vi "main.vi"() -> ()   [LabVIEW 2021]
uses:
  Controls/App Data.ctl
  Controls/UI References.ctl
  <extravilib>/ChannelInstances/Stream-c(dbl,dbl)/Read With Abort.vi
  <extravilib>/ChannelInstances/Stream-c(dbl,dbl)/Write With Abort.vi
  <extravilib>/ChannelInstances/Stream-c(dbl,dbl)/EndpointRead.vi
  <extravilib>/ChannelInstances/Stream-c(dbl,dbl)/Endpoint.vi
  <extravilib>/ChannelInstances/Event Messenger-c(str,var)/Instantiate.vi
  <extravilib>/ChannelInstances/Event Messenger-c(str,var)/))Channel.vi
  <extravilib>/ChannelInstances/Stream-c(dbl,dbl)/Instantiate.vi
  <extravilib>/ChannelInstances/Stream-c(dbl,dbl)/)Channel.vi
  <resource>/ChannelSupport/_ChannelSupport/WaitIfNeeded.vi
  <vilib>/Instr/_visa.llb/VISA Configure Serial Port (Instr).vi
  <extravilib>/ChannelInstances/Stream-c(dbl,dbl).lvlib
  <extravilib>/ChannelInstances/Event Messenger-c(str,var).lvlib
panel:
  in  "Confirm":bool
  in  "Start":bool
  out "File Path":path
  out "Recording?":bool
  in  "Record?":bool
  out "XY Graph":cluster{"X":dbl, "Y":dbl}[](graph)
  out "Strain":dbl
  out "Time":dbl
  in  "VISA resource name":refnum<visa-resource-name>
  in  "Stop":bool
  # "Select the VISA resource name before starting the application, you can choose to record to a file at any time using the checkbox. Data acquisition begins after you press Start."
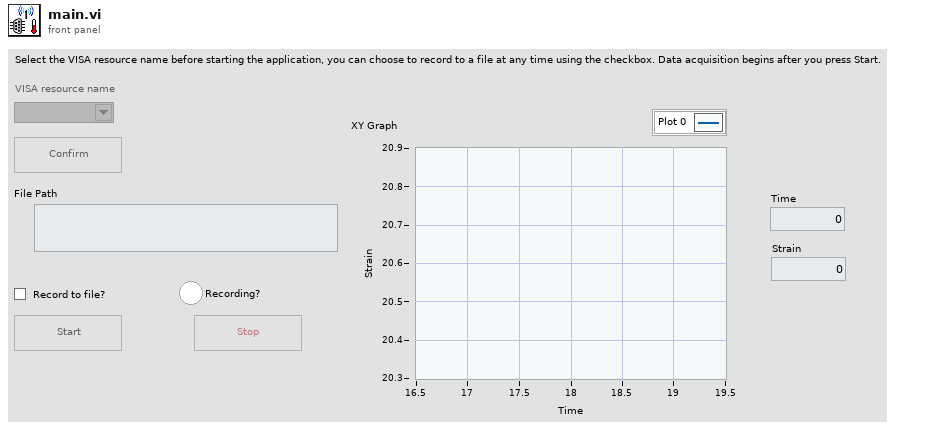
[diagram p1: front panel]
types:
  T1 = typedef "UI References.ctl" = cluster{"VISA resource name":refnum<vi>, "Confirm":refnum<vi>, "Start":refnum<vi>, "Stop":refnum<vi>, "Record?":refnum<vi>, "Recording?":refnum<vi>, "XY Graph":refnum<vi>}
  T2 = typedef "App Data.ctl" = cluster{"VISA resource name":refnum<visa-resource-name>, "File ref":refnum<file>}
  T3 = typedef "Event Messenger-c(str,var).lvlib/))Channel.ctl" = refnum<queue>
  T4 = typedef "Stream-c(dbl,dbl).lvlib/)Channel.ctl" = refnum<queue>
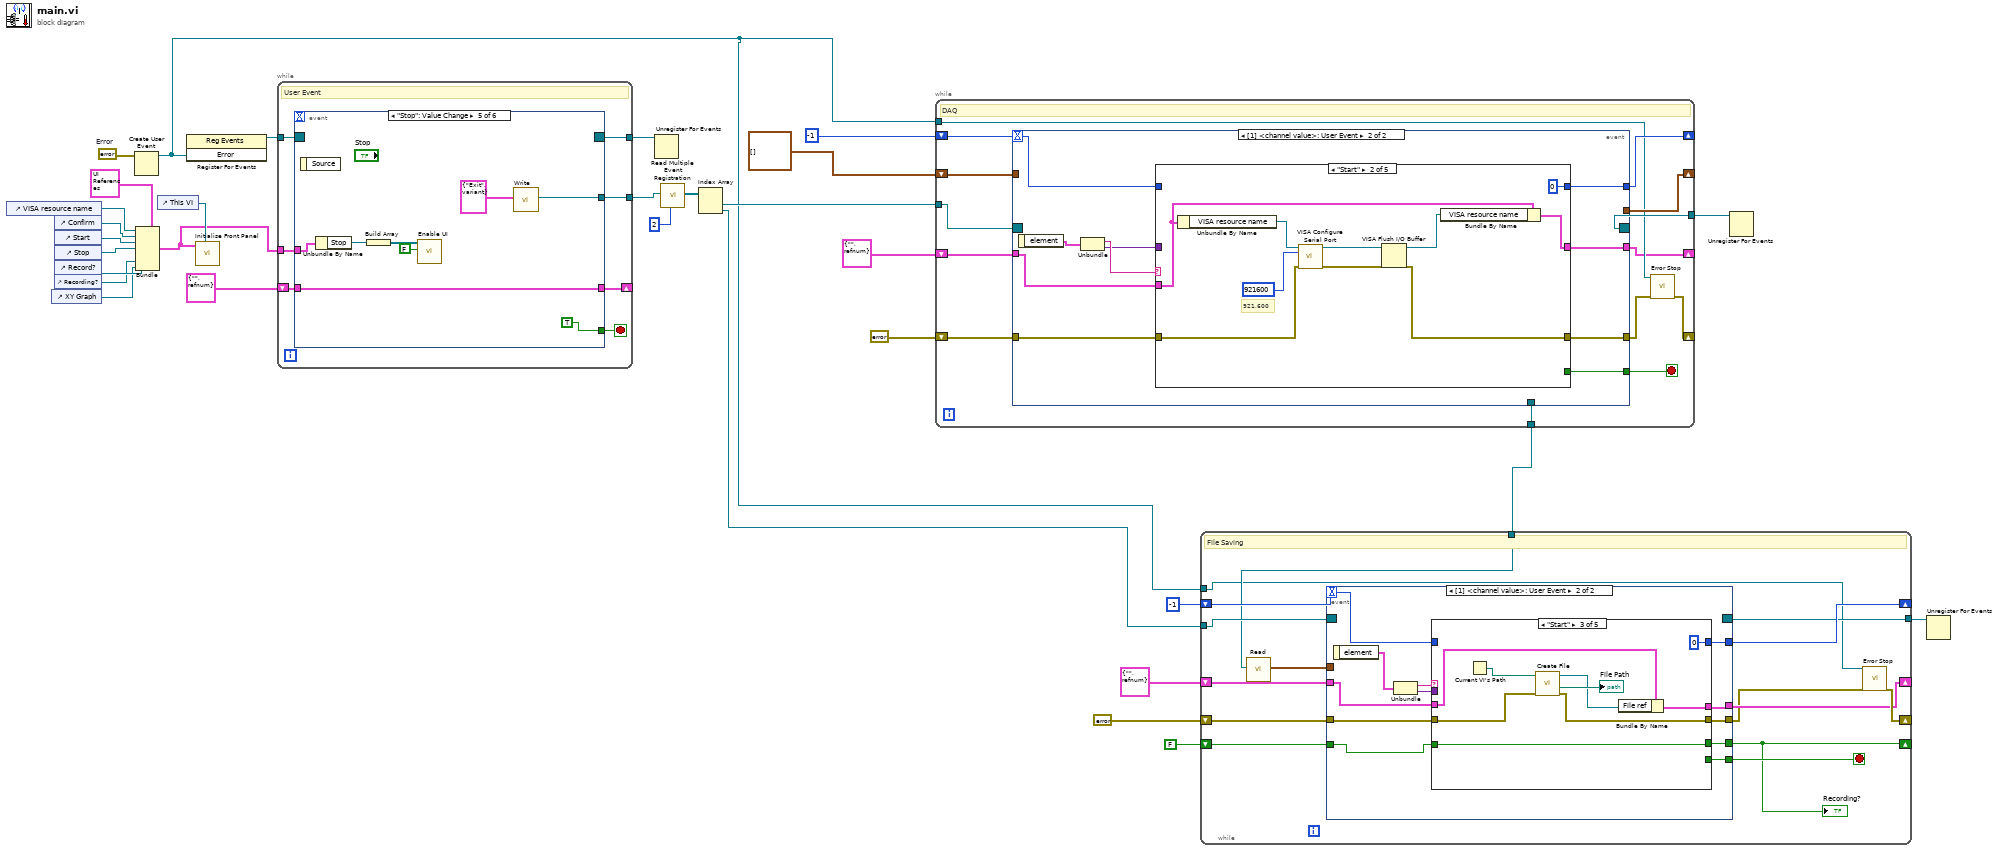
[diagram p0: block diagram]
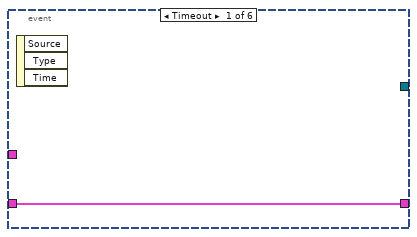
[diagram p2: hidden frame]
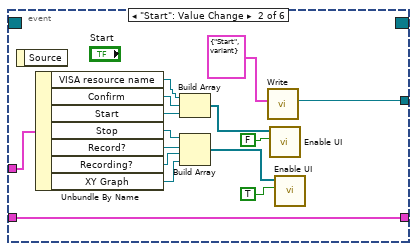
[diagram p3: hidden frame]
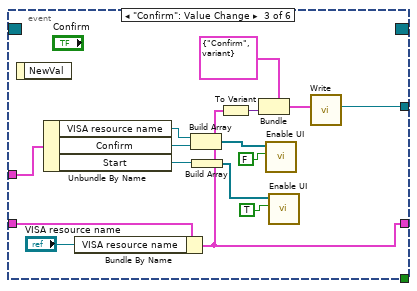
[diagram p4: hidden frame]
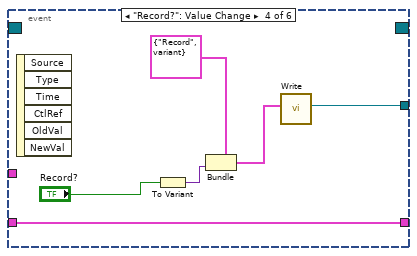
[diagram p5: hidden frame]
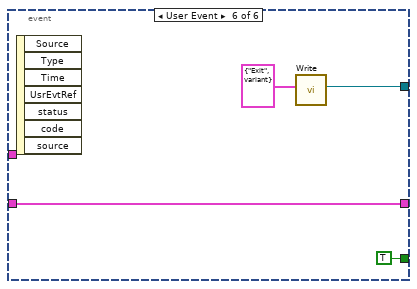
[diagram p6: hidden frame]
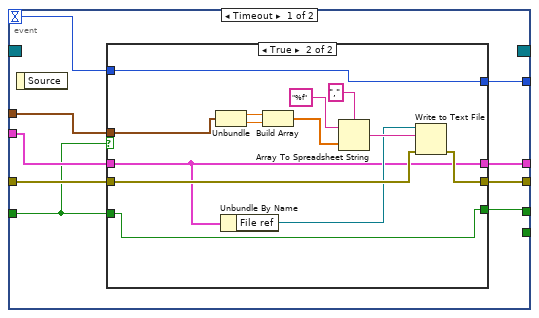
[diagram p7: hidden frame]
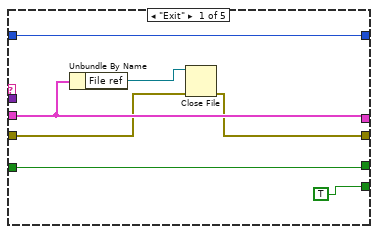
[diagram p9: hidden frame]
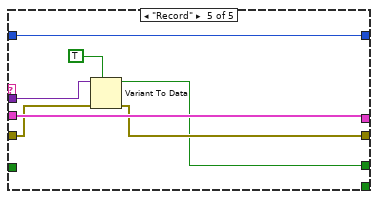
[diagram p12: hidden frame]
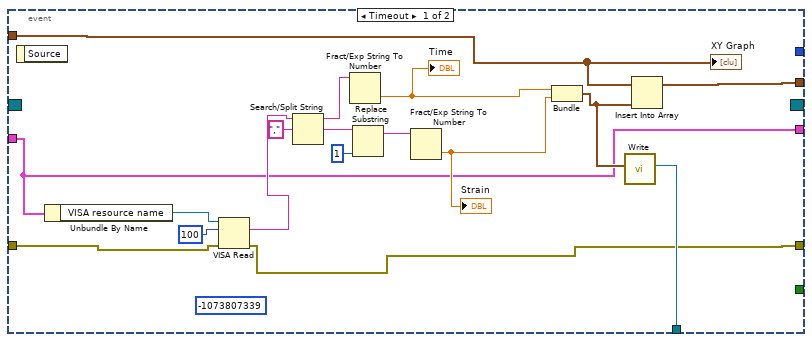
[diagram p13: hidden frame]
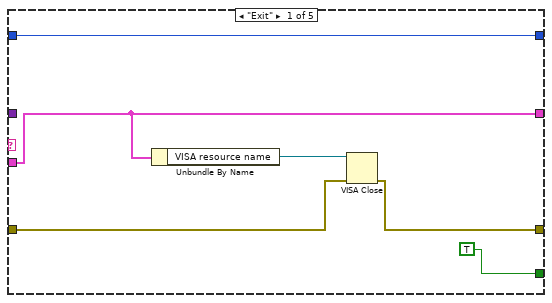
[diagram p14: hidden frame]
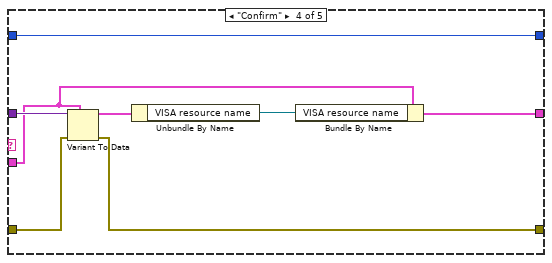
[diagram p16: hidden frame]
diagram:
  w23 = errorcluster {"status"=FALSE, "code"=0, "source"=""}  # Error
  n1 = control-ref of="VISA resource name"() -> (w4:refnum<vi>)
  n2 = control-ref of="XY Graph"() -> (w6:refnum<vi>)
  n3 = control-ref of="Confirm"() -> (w3:refnum<vi>)
  n4 = control-ref of="Start"() -> (w11:refnum<vi>)
  n5 = control-ref of="Stop"() -> (w10:refnum<vi>)
  n6 = control-ref of="Record?"() -> (w9:refnum<vi>)
  n7 = control-ref of="Recording?"() -> (w7:refnum<vi>)
  n8 = Create User Event(user event datatype=w23) -> (user event=w22:refnum<user-event>)  [unwired: 1 in, 1 out]
  n9 = Bundle(cluster=T1 {"VISA resource name"=refnum, "Confirm"=refnum, "Start"=refnum, "Stop"=refnum, "Record?"=refnum, "Recording?"=refnum, "XY Graph"=refnum} ("UI Ref"), "VISA resource name"=w4, "Confirm"=w3, "Start"=w11, "Stop"=w10, "Record?"=w9, "Recording?"=w7, "XY Graph"=w6) -> (w5:T1)
  n10 = control-ref of="This VI"() -> (w8:refnum<vi>)
  n11 = register-events(w22) -> (reference out=w29:refnum<event-registration>)  [unwired: 2 in, 1 out]
  n12 = call "Initialise Front Panel.vi"("This VI"=w8, "UI Ref"=w5) -> ()  [unwired: 9 in, 1 out]
  n13 = while {
    tunnel: w29 -> [w38]
    tunnel: [w37] -> w28
    tunnel: [w36] -> w27
    shift-right: [w34] -> _
    shift-left: T2 {"VISA resource name"="", "File ref"=refnum} ("App Data") -> [w33]
    tunnel: w5 -> [w32]
    stop <- w35 stop-if-true
    # "User Event"
    n14 = event shown="[4] \"Stop\": Value Change" {
      selector: w38 -> [_ _ _ _ _ _]
      dyn-events: [_ _ _ _ _ _] -> w37
      timeout: _ -> [_ _ _ _ _ _]
      tunnel: [_ w54 w68 w75 w81 w86] -> w36
      tunnel: [_ _ _ _ TRUE TRUE] -> w35
      tunnel: [w39 w52 w66 w74 w80 w84] -> w34
      tunnel: w33 -> [w39 w52 w67 w74 w80 w84]
      tunnel: w32 -> [_ w51 w65 _ w79 _]
      event Timeout {
        n15 = event-data() -> ()  [unwired: 1 in, 3 out]
      }
      event "Start": Value Change {
        n16 = event-data() -> ()  [unwired: 1 in, 1 out]
        n17 = Unbundle By Name(w51) -> ("VISA resource name"=w40:refnum<vi>, "Confirm"=w42:refnum<vi>, "Start"=w50:refnum<vi>, "Stop"=w41:refnum<vi>, "Record?"=w49:refnum<vi>, "Recording?"=w48:refnum<vi>, "XY Graph"=w47:refnum<vi>)
        n18 = Build Array(w40, w42, w50) -> (w46:refnum<vi>[])
        n19 = Build Array(w41, w49, w48, w47) -> (w45:refnum<vi>[])
        n20 = call <extravilib>:"Write.vi"("element"=cluster{string, variant} {"Start", variant}) -> ("channel"=w54:T3)  [unwired: 9 in, 1 out]
        n21 = call "Enable UI.vi"("Enable?"=FALSE, "output cluster"=w46) -> ()  [unwired: 9 in, 1 out]
        n22 = call "Enable UI.vi"("Enable?"=TRUE, "output cluster"=w45) -> ()  [unwired: 9 in, 1 out]
      }
      event "Confirm": Value Change {
        n23 = event-data() -> ()  [unwired: 1 in, 1 out]
        n24 = Unbundle By Name(w65) -> ("VISA resource name"=w56:refnum<vi>, "Confirm"=w64:refnum<vi>, "Start"=w63:refnum<vi>)
        n25 = Bundle By Name(cluster=w67, "VISA resource name"="VISA resource name") -> (w66:T2)
        n26 = Build Array(w56, w64) -> (w60:refnum<vi>[])
        n27 = Build Array(w63) -> (w59:refnum<vi>[])
        n28 = To Variant(anything=w66) -> (Variant=w69:variant)
        n29 = Bundle(cluster=cluster{string, variant} {"Confirm", variant}, w69) -> (w61:cluster{string, variant})  [unwired: 1 in]
        n30 = call "Enable UI.vi"("Enable?"=FALSE, "output cluster"=w60) -> ()  [unwired: 9 in, 1 out]
        n31 = call "Enable UI.vi"("Enable?"=TRUE, "output cluster"=w59) -> ()  [unwired: 9 in, 1 out]
        n32 = call <extravilib>:"Write.vi"("element"=w61) -> ("channel"=w68:T3)  [unwired: 9 in, 1 out]
      }
      event "Record?": Value Change {
        n33 = event-data() -> ()  [unwired: 1 in, 6 out]
        n34 = To Variant(anything="Record?") -> (Variant=w72:variant)
        n35 = Bundle(cluster=cluster{string, variant} {"Record", variant}, w72) -> (w70:cluster{string, variant})  [unwired: 1 in]
        n36 = call <extravilib>:"Write.vi"("element"=w70) -> ("channel"=w75:T3)  [unwired: 9 in, 1 out]
      }
      event "Stop": Value Change {
        n37 = event-data() -> ()  [unwired: 1 in, 1 out]
        n38 = Unbundle By Name(w79) -> ("Stop"=w78:refnum<vi>)
        n39 = Build Array(w78) -> (w77:refnum<vi>[])
        n40 = call "Enable UI.vi"("Enable?"=FALSE, "output cluster"=w77) -> ()  [unwired: 9 in, 1 out]
        n41 = call <extravilib>:"Write.vi"("element"=cluster{string, variant} {"Exit", variant}) -> ("channel"=w81:T3)  [unwired: 9 in, 1 out]
      }
      event User Event {
        n42 = event-data() -> ()  [unwired: 1 in, 7 out]
        n43 = call <extravilib>:"Write.vi"("element"=cluster{string, variant} {"Exit", variant}) -> ("channel"=w86:T3)  [unwired: 9 in, 1 out]
      }
    }
  }
  n44 = Unregister For Events(event registration refnum=w28) -> ()  [unwired: 1 in, 1 out]
  n45 = call <extravilib>:"Read Multiple Event Registration.vi"("number of event structures"=u16 2, "channel"=w27) -> ("event registration refnums"=w18:refnum<event-registration>[])  [unwired: 9 in]
  n46 = Index Array(array=w18) -> (element #1=w26:refnum<event-registration>, element #2=w24:refnum<event-registration>)  [unwired: 2 in]
  n47 = while {
    shift-right: [w101] -> _
    shift-left: cluster{dbl, dbl}[] [] -> [w100]
    tunnel: [w99] -> w30
    tunnel: w26 -> [w98]
    tunnel: [w97] -> w25
    tunnel: w22 -> [w93]
    shift-right: [w94] -> _
    shift-left: -1 -> [w95]
    shift-right: [w88] -> _
    shift-left: T2 {"VISA resource name"="", "File ref"=refnum} ("App Data") -> [w89]
    shift-right: [w92] -> _
    shift-left: errorcluster {"status"=FALSE, "code"=0, "source"=""} ("error in (no error)") -> [w90]
    stop <- w96 stop-if-true
    # "DAQ"
    n48 = event shown="[1] <channel value>: User Event" {
      selector: w98 -> [_ _]
      dyn-events: [_ _] -> w97
      timeout: w95 -> [_ w125]
      tunnel: [w118 _] -> w101
      tunnel: w100 -> [w117 _]
      tunnel: [w116 _] -> w99
      tunnel: [w102 w122] -> w91
      tunnel: [_ w126] -> w96
      tunnel: [_ w124] -> w94
      tunnel: w90 -> [w103 w121]
      tunnel: w89 -> [w104 w120]
      tunnel: [w104 w119] -> w88
      event Timeout {
        (unwired) -1073807339 ("specific error code to clear (0: all)")
        n49 = event-data() -> ()  [unwired: 1 in, 1 out]
        n50 = Unbundle By Name(w104) -> ("VISA resource name"=w105:refnum<visa-resource-name>)
        n51 = VISA Read(VISA resource name=w105, byte count=u32 100, error in (no error)=w103) -> (read buffer=w113:string, error out=w102:errorcluster)  [unwired: 2 out]
        n52 = Search/Split String(string=w113, search string/char (-)=",") -> (substring before match=w112:string, match + rest of string=w111:string)  [unwired: 1 in, 1 out]
        n53 = Fract/Exp String To Number(string=w112) -> (number=w108:dbl)  [unwired: 3 in, 1 out]
        "Time" <- w108
        n54 = Replace Substring(2:1 ("length (len. of substring)"), 5:w111) -> (1:w109:string)  [unwired: 2 in, 1 out]
        n55 = Fract/Exp String To Number(string=w109) -> (number=w107:dbl)  [unwired: 3 in, 1 out]
        "Strain" <- w107
        n56 = Bundle(w108, w107) -> (w106:cluster{dbl, dbl})  [unwired: 1 in]
        n57 = call <extravilib>:"Write.vi"("element"=w106) -> ("channel"=w116:T4)  [unwired: 8 in, 2 out]
        n58 = Insert Into Array(array=w117, new element=w106) -> (w118:cluster{dbl, dbl}[])  [unwired: 1 in]
        "XY Graph" <- w117
      }
      event User Event {
        n59 = event-data() -> ("element"=w128:cluster{string, "Data":variant})  [unwired: 1 in]
        n60 = Unbundle(w128) -> (w127:string, "Data"=w123:variant)
        n61 = case shown="\"Start\"" w127 {
          tunnel: [TRUE _ _ _ _] -> w126
          tunnel: w125 -> [w129 _ w147 w153 w158]
          tunnel: [w129 0 w147 w153 w158] -> w124
          tunnel: w123 -> [_ _ _ w155 _]
          tunnel: [w130 w138 w145 w148 w157] -> w122
          tunnel: w121 -> [w131 w139 w145 w154 w157]
          tunnel: w120 -> [w133 w137 w146 w151 w156]
          tunnel: [w133 w135 w146 w149 w156] -> w119
          frame "Exit" {
            n62 = Unbundle By Name(w133) -> ("VISA resource name"=w132:refnum<visa-resource-name>)
            n63 = VISA Close(VISA resource name=w132, error in (no error)=w131) -> (error out=w130:errorcluster)
          }
          frame "Start" {
            # "921,600"
            n64 = Unbundle By Name(w137) -> ("VISA resource name"=w140:refnum<visa-resource-name>)
            n65 = call-poly "VISA Configure Serial Port"("VISA resource name"=w140, "baud rate (9600)"=u32 921600, "error in (no error)"=w139) -> ("VISA resource name out"=w141:refnum<visa-resource-name>, "error out"=w142:errorcluster)  [unwired: 11 in]
            n66 = VISA Flush I/O Buffer(VISA resource name=w141, error in (no error)=w142) -> (VISA resource name out=w136:refnum<visa-resource-name>, error out=w138:errorcluster)  [unwired: 1 in]
            n67 = Bundle By Name(cluster=w137, "VISA resource name"=w136) -> (w135:T2)
          }
          frame "Record" {
          }
          frame "Confirm" {
            n68 = Variant To Data(error in=w154, type=w151, Variant=w155) -> (data=w152:T2, error out=w148:errorcluster)
            n69 = Unbundle By Name(w152) -> ("VISA resource name"=w150:refnum<visa-resource-name>)
            n70 = Bundle By Name(cluster=w151, "VISA resource name"=w150) -> (w149:T2)
          }
          frame Default {
          }
        }
      }
    }
    n71 = call "Error Stop.vi"("error in"=w91, "user event"=w93) -> ("error out"=w92:errorcluster)  [unwired: 9 in]
  }
  n72 = while {
    shift-right: [w163] -> _
    shift-left: errorcluster {"status"=FALSE, "code"=0, "source"=""} ("error in (no error)") -> [w173]
    tunnel: w30 -> [w166]
    tunnel: w24 -> [w172]
    tunnel: w22 -> [w164]
    shift-right: [w170] -> _
    shift-left: -1 -> [w171]
    shift-right: [w159] -> _
    shift-left: FALSE -> [w168]
    tunnel: [w165] -> w19
    shift-right: [w161] -> _
    shift-left: T2 {"VISA resource name"="", "File ref"=refnum} ("App Data") -> [w162]
    stop <- w169 stop-if-true
    # "File Saving"
    n73 = call <extravilib>:"Read.vi"("channel"=w166) -> ("element"=w167:cluster{dbl, dbl})  [unwired: 6 in, 4 out]
    n74 = event shown="[1] <channel value>: User Event" {
      selector: w172 -> [_ _]
      dyn-events: [_ _] -> w165
      timeout: w171 -> [w176 w209]
      tunnel: w173 -> [w182 w204]
      tunnel: [w179 w203] -> w160
      tunnel: [w175 w208] -> w170
      tunnel: [_ w207] -> w169
      tunnel: [w181 w206] -> w159
      tunnel: w168 -> [w174 w205]
      tunnel: w167 -> [w180 _]
      tunnel: w162 -> [w178 w202]
      tunnel: [w177 w201] -> w161
      event Timeout {
        n75 = event-data() -> ()  [unwired: 1 in, 1 out]
        n76 = case shown="True" w174 {
          tunnel: [w186 w191] -> w179
          tunnel: w182 -> [w186 w192]
          tunnel: [w183 w187] -> w181
          tunnel: w180 -> [_ w194]
          tunnel: w178 -> [w185 w189]
          tunnel: [w185 w189] -> w177
          tunnel: w176 -> [w184 w188]
          tunnel: [w184 w188] -> w175
          tunnel: w174 -> [w183 w187]
          frame False {
          }
          frame True {
            n77 = Unbundle(w194) -> (w199:dbl, w198:dbl)
            n78 = Unbundle By Name(w189) -> ("File ref"=w190:refnum<file>)
            n79 = Build Array(w199, w198) -> (w195:dbl[])
            n80 = Array To Spreadsheet String(delimiter (Tab)=",", array=w195, 3:"%f" ("format string")) -> (spreadsheet string=w193:string)
            n81 = Write to Text File(file (use dialog)=w190, text=w193, error in=w192) -> (error out=w191:errorcluster)  [unwired: 1 in, 2 out]
          }
        }
      }
      event User Event {
        n82 = event-data() -> ("element"=w211:cluster{string, "Data":variant})  [unwired: 1 in]
        n83 = Unbundle(w211) -> (w210:string, "Data"=w200:variant)
        n84 = case shown="\"Start\"" w210 {
          tunnel: w209 -> [w217 w222 _ w235 w241]
          tunnel: [w217 w222 0 w235 w241] -> w208
          tunnel: [TRUE _ _ _ _] -> w207
          tunnel: [w212 w219 w227 w232 w236] -> w206
          tunnel: w205 -> [w212 w219 w227 w232 _]
          tunnel: w204 -> [w214 w220 w229 w233 w238]
          tunnel: [w213 w220 w228 w233 w237] -> w203
          tunnel: w202 -> [w216 w221 w226 w234 w242]
          tunnel: [w216 w221 w224 w234 w242] -> w201
          tunnel: w200 -> [_ _ _ _ w239]
          frame "Exit" {
            n85 = Unbundle By Name(w216) -> ("File ref"=w215:refnum<file>)
            n86 = Close File(refnum=w215, error in=w214) -> (error out=w213:errorcluster)  [unwired: 1 out]
          }
          frame Default {
          }
          frame "Start" {
            n87 = Current VI's Path() -> (path=w231:path)
            n88 = call "Create File.vi"("error in"=w229, "Root Path"=w231) -> ("error out"=w228:errorcluster, "File path out"=→"File Path":path, "refnum out"=w225:refnum<file>)  [unwired: 7 in]
            n89 = Bundle By Name(cluster=w226, "File ref"=w225) -> (w224:T2)
          }
          frame "Confirm" {
          }
          frame "Record" {
            n90 = Variant To Data(error in=w238, type=TRUE, Variant=w239) -> (data=w236:bool, error out=w237:errorcluster)
          }
        }
      }
    }
    "Recording?" <- w159
    n91 = call "Error Stop.vi"("error in"=w160, "user event"=w164) -> ("error out"=w163:errorcluster)  [unwired: 9 in]
  }
  n92 = Unregister For Events(event registration refnum=w25) -> ()  [unwired: 1 in, 1 out]
  n93 = Unregister For Events(event registration refnum=w19) -> ()  [unwired: 1 in, 1 out]
